vi "CRYStep Setup Replace.vi"(8 "sOption Etc":string, 9 "Current Step Setup VI No":i32, 10 "sOption":string, 11 "Category":string) -> ()   [LabVIEW 2013]
uses:
  CRYStepSetup/CRYStepSetup Global.vi
  CRYCurveLibrary/Global/CRYCurve Library Global.vi
  CRYProject Editor Global.vi
  user32.dll
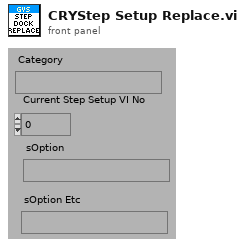
[diagram p1: front panel]
types:
  T1 = typedef "CRYTS.ctl" = cluster{"No.TS":u16, "TS File Path":path, "TS Name":string, "EditStepName":string, "Steps":T2[], "New State":bool, "Change State":bool, "Flattened CurveLib Data":string, "Document Data":string, "EditStepNo":u16, "Operator Start File":string, "Sequence Type":string, "Sequence Language":string}
  T2 = typedef "CRYStep.ctl" = cluster{"No.VI":i32, "Category":string, "StepName":string, "Seq setup flattened":string, "Comment":string, "Steps config.":bool[], "Jump config":i32[], "Start":dbl, "Increment":dbl, "Name":string, "Unit":string, "Y data":u16, "Y prefix":string, "Y dB ref":dbl, "Y unit":string, "Repeat State Array":cluster{"Start":dbl, "Increment":dbl, "Count":i32, "Num":i32}[]}
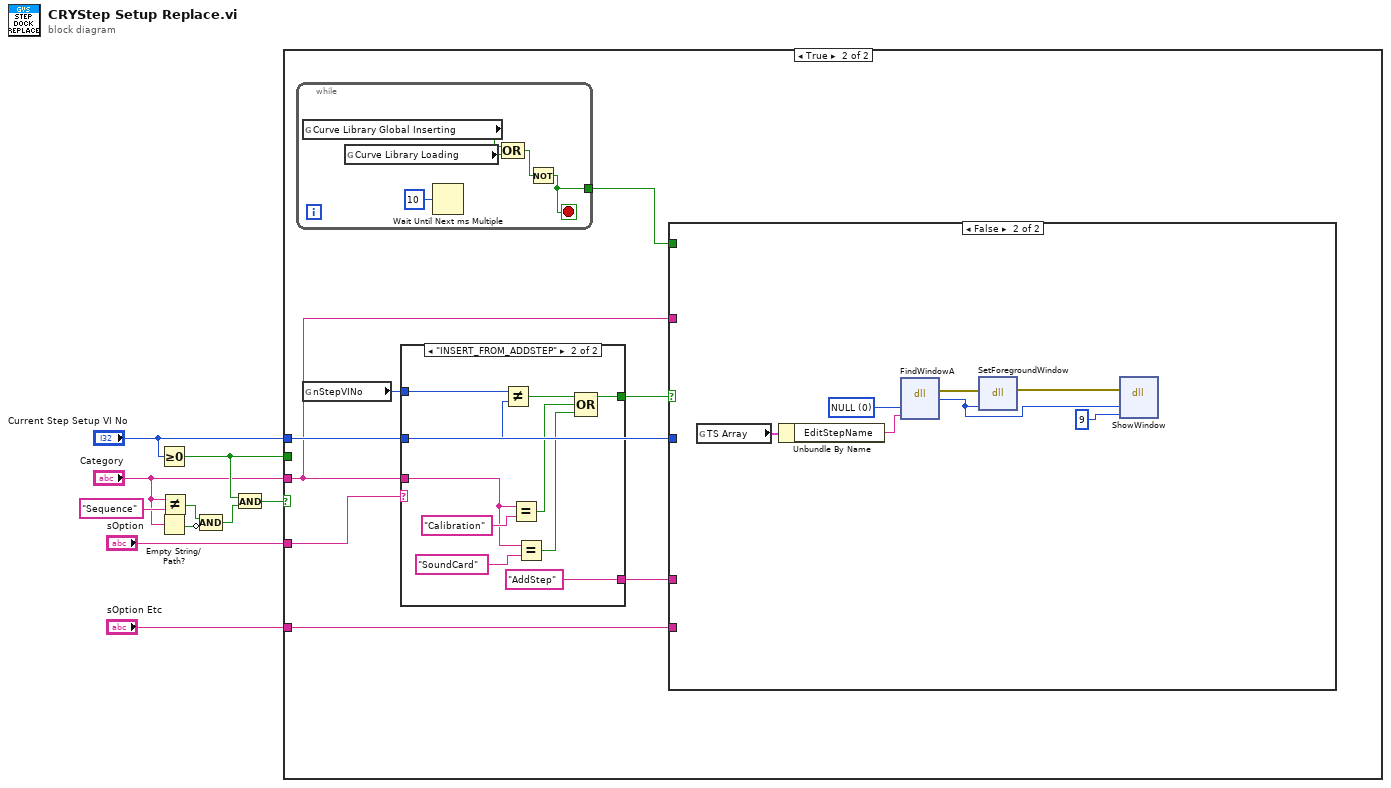
[diagram p0: block diagram]
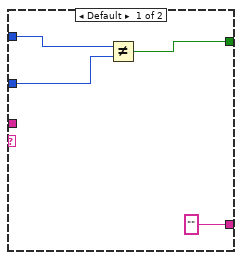
[diagram p3: hidden frame]
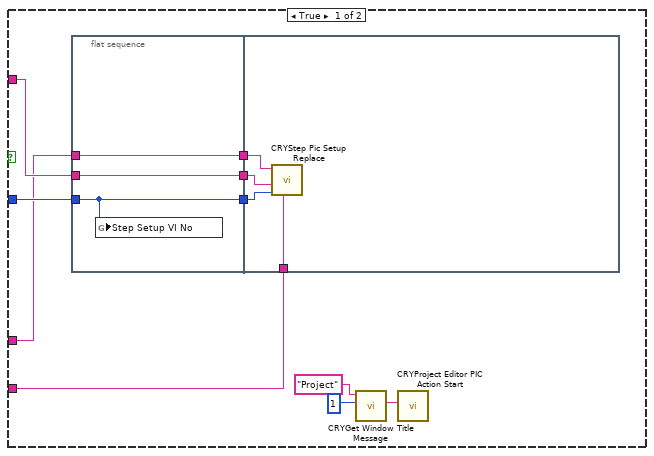
[diagram p4: hidden frame]
diagram:
  n1 = Greater Or Equal To 0?(x="Current Step Setup VI No") -> (x >= 0?=w7:bool)
  n2 = Empty String/Path?(string/path="Category") -> (empty?=w3:bool)
  n3 = Not Equal?(x="Category", y="Sequence") -> (x != y?=w4:bool)
  n4 = Compound Arithmetic op=AND(w4, invert w3) -> (w2:bool)
  n5 = And(x=w7, y=w2) -> (x .and. y?=w8:bool)
  n6 = case shown="True" w8 {
    tunnel: "Current Step Setup VI No" -> [_ w18]
    tunnel: "Category" -> [_ w14]
    tunnel: "sOption" -> [_ w13]
    tunnel: w7 -> [_ _]
    tunnel: "sOption Etc" -> [_ w11]
    frame False {
    }
    frame True {
      n7 = while {
        tunnel: [w33] -> w17
        stop <- w33 stop-if-true
        n8 = global read "CRYCurve Library Global.vi" "Curve Library Global Inserting"() -> (w34:bool)
        n9 = global read "CRYCurve Library Global.vi" "Curve Library Loading"() -> (w35:bool)
        n10 = Wait Until Next ms Multiple(millisecond multiple=u32 10 ("milliseconds to wait")) -> ()  [unwired: 1 out]
        n11 = Compound Arithmetic op=OR(w34, w35) -> (w36:bool)
        n12 = Not(x=w36) -> (.not. x?=w33:bool)
      }
      n13 = global read "CRYStepSetup Global.vi" "nStepVINo"() -> (w16:i32)
      n14 = case shown="\"INSERT_FROM_ADDSTEP\"" w13 {
        tunnel: w18 -> [w21 w32]
        tunnel: w16 -> [w22 w30]
        tunnel: w14 -> [_ w28]
        tunnel: [w20 w26] -> w15
        tunnel: ["" ("sOption") "AddStep" ("sOption")] -> w12
        frame Default {
          n15 = Not Equal?(x=w22, y=w21) -> (x != y?=w20:bool)
        }
        frame "INSERT_FROM_ADDSTEP" {
          n16 = Not Equal?(x=w30, y=w32) -> (x != y?=w31:bool)
          n17 = Equal?(x=w28, y="Calibration" ("Down Step Name")) -> (x = y?=w25:bool)
          n18 = Equal?(x=w28, y="SoundCard" ("Down Step Name")) -> (x = y?=w24:bool)
          n19 = Compound Arithmetic op=OR(w31, w25, w24) -> (w26:bool)
        }
      }
      n20 = case shown="False" w15 {
        tunnel: w18 -> [w47 _]
        tunnel: w17 -> [_ _]
        tunnel: w14 -> [w46 _]
        tunnel: w12 -> [w39 _]
        tunnel: w11 -> [w38 _]
        frame True {
          n21 = flat-sequence {
            tunnel: w46 -> [w50]
            tunnel: w47 -> [w49]
            tunnel: [w49] -> w45
            tunnel: [w50] -> w44
            tunnel: [w48] -> w40
            tunnel: w39 -> [w48]
            tunnel: w45 -> [w53]
            tunnel: w44 -> [w54]
            tunnel: w40 -> [w52]
            tunnel: w38 -> [w51]
            frame #0 {
              n22 = global write "CRYProject Editor Global.vi" "Step Setup VI No"(w49) -> ()
            }
            frame #1 {
              n23 = call "CRYStep Pic Setup Replace .vi"("sOption Etc"=w51, "nData"=w53, "sStepName"=w54, "sOption"=w52) -> ()  [unwired: 7 in, 1 out]
            }
          }
          n24 = call "CRYGet Window Title Message.vi"("No"=1 ("Error No"), "Kind"="Project") -> ("Unicode String"=w42:string)  [unwired: 4 in, 5 out]
          n25 = call "CRYProject Editor PIC Action Start.vi"("sData"=w42) -> ()  [unwired: 11 in]
        }
        frame False {
          w61 = 0 items=["NULL"]
          n26 = global read "CRYProject Editor Global.vi" "TS Array"() -> (w60:T1)
          n27 = Unbundle By Name(w60) -> ("EditStepName"=w59:string)
          n28 = dll-call lib="user32.dll" fn="FindWindowA" label="FindWindow"("lpszClassName"=w61, "lpszWindowName"=w59) -> (error out=w57:errorcluster, "hWnd"=w55:u32)  [unwired: 4 in, 2 out]
          n29 = dll-call lib="user32.dll" fn="SetForegroundWindow"(error in=w57, "Handle"=w55) -> (error out=w56:errorcluster)  [unwired: 3 in, 2 out]
          n30 = dll-call lib="user32.dll" fn="ShowWindow"(error in=w56, "Handle"=w55, "nCmdShow"=9) -> ()  [unwired: 4 in, 3 out]
        }
      }
    }
  }
